vi "Output StatusMod2.vi"(8 "error in (no error)":errorcluster, 11 "Refnum in":refnum<k20>) -> (0 "error out":errorcluster, 2 "status":T1, 3 "Refnum out":refnum<k20>)   [LabVIEW 2017]
uses:
  <vilib>/Utility/error.llb/Error Cluster From Error Code.vi
  <vilib>/rvi/errors/niLvFpgaAdjustHostInterfaceError.vi
  <vilib>/rvi/interface/nirviReadWriteControl/nirviReadWriteControl.xnode
  NiFpgaLv.dll
  <vilib>/rvi/interface/Simulation/niFpgaSimulationCallBeginRW.vi
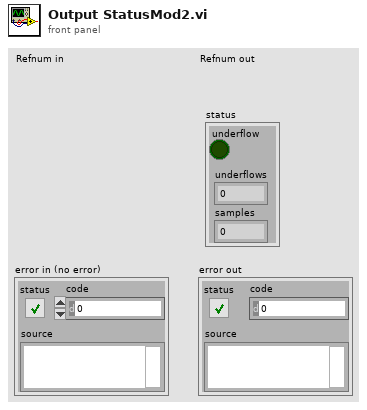
[diagram p1: front panel]
types:
  T1 = cluster{"underflow":bool, "underflows":u32, "samples":u32}
  T2 = cluster{"streaming output.underflow":bool, "streaming output.underflows":u32, "streaming output.samples processed":u32}
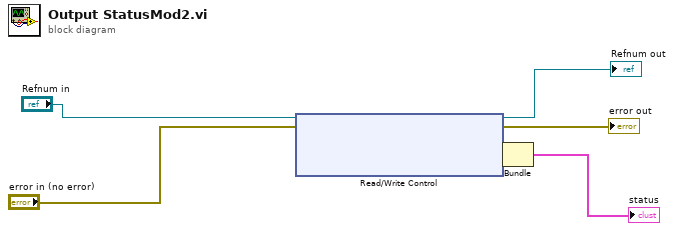
[diagram p0: block diagram]
diagram:
  n1 = xnode "Read/Write Control"("FPGA VI Reference In"="Refnum in", "error in"="error in (no error)") -> ("FPGA VI Reference Out"=→"Refnum out":refnum<k20>, "error out"=→"error out":errorcluster, "streaming output.underflow"=w2:bool, "streaming output.underflows"=w3:u32, "streaming output.samples processed"=w4:u32)
  n2 = Bundle("streaming output.underflow"=w2, "streaming output.underflows"=w3, "streaming output.samples processed"=w4) -> (→"status":T2)  [unwired: 1 in]
